vi "Draw Circle.vi"() -> ()   [LabVIEW 2016]
uses:
  Classes/Controller/Motion/A3200 Folder/A3200.lvclass
panel:
  in  "XY End":dbl[](array[numeric])=[410.0, 810.0] format="%#_13g"
  in  "Speed 2":dbl=20.0 format="%#_13g"
  in  "radius":dbl=20.0 format="%#_13g"
  in  "Direction":u16(ring)=1 items=["Clockwise", "Counter-clockwise"]
  in  "XY Center":dbl[](array[numeric])=[10.0, 0.0]
  in  "XY End 2":dbl[](array[numeric])=[400.0, 800.0]
  in  "Speed 3":dbl=20.0
  in  "Direction 2":u16(ring)=1 items=["Clockwise", "Counter-clockwise"]
  in  "Draw circle method":string(combo)="Circular"
  in  "XY":dbl[](array[numeric])=[400.0, 800.0]
  in  "Speed":dbl=40.0
  # "Circular Radius"
  # "* Draw pattern with circle radius specified, then the path would be constructed with the initial position and the end position. \n* You use this function if you don't want to calculate the circle center, you just want to draw an arc\n* You cannot draw over half circle with this function\n\n1. An arc with radius 20\n    a. radius: (20, 0)\n    b. XY End: (410, 810)"
  # "Circular"
  # "* Draw pattern with circle center specified, then the circle would be constructed with the initial position and the center position. \n* Circle Center is relative position to the initial position\n* End point could be on any position on the circle\n\n1. Full Circle with center at (410, 800)\n    a. XY Center: (10, 0)\n    b. XY End: (400, 800)\n2. Half Circle with center at (400, 810)\n    a. XY Center: (0, 10) \n    b. XY End: (400, 820)"
  # "1. This example shows how to draw a circle/arc on the XY plane  \n2. There are two methods \"Circular\" & \"Circular Radius\n3. \"Circular\" method is more commonly used \n4. Both two functions need to move gantry head to initial point of your circle/arc first"
  # "Move To Initial"
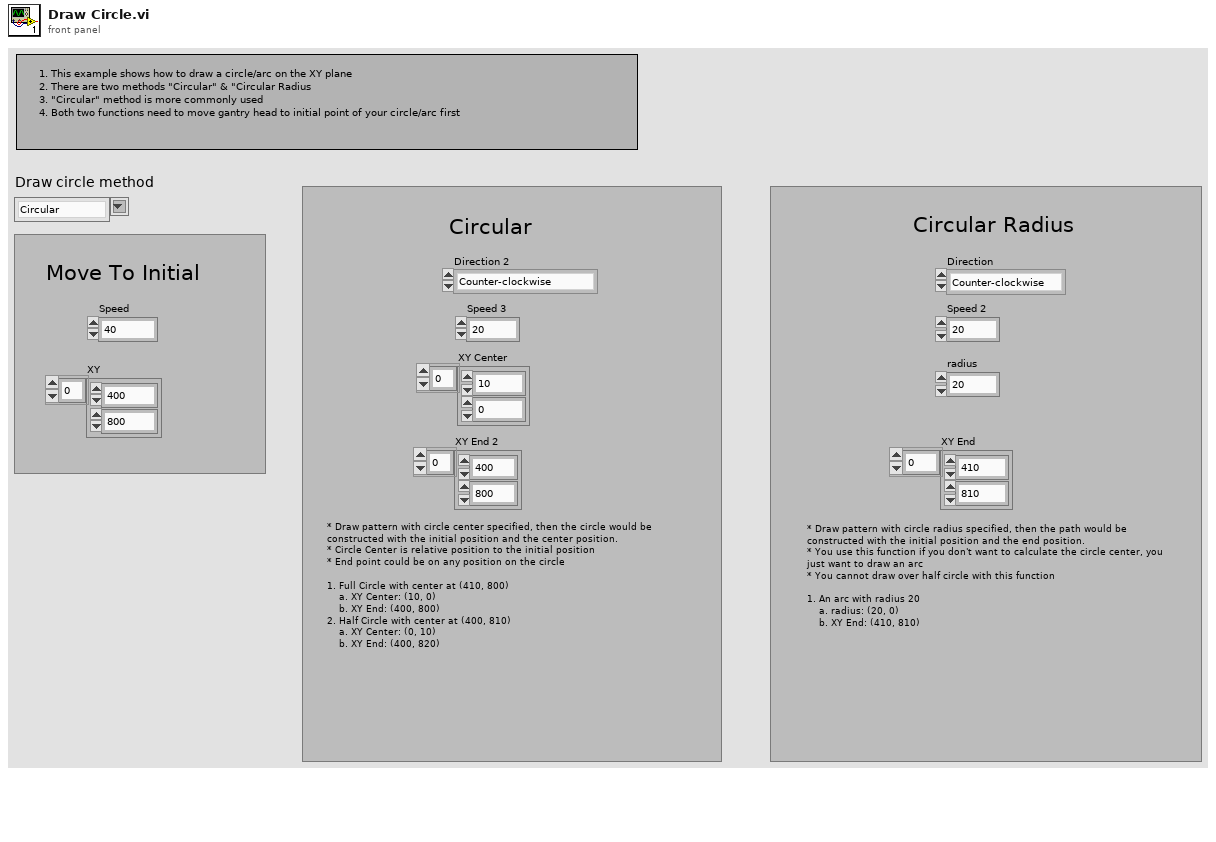
[diagram p1: front panel]
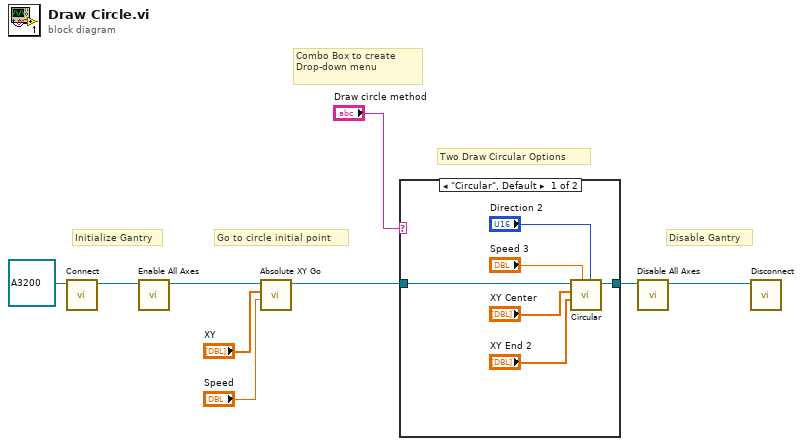
[diagram p0: block diagram]
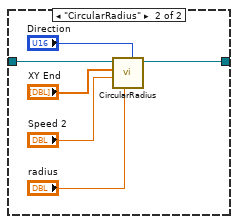
[diagram p2: hidden frame]
diagram:
  # "Disable Gantry"
  # "Go to circle initial point"
  # "Initialize Gantry"
  # "Combo Box to create Drop-down menu"
  # "Two Draw Circular Options"
  n1 = call-dynamic "Connect.vi"("Gantry in"=refnum<class "A3200.lvclass"> refnum ("A3200.lvclass")) -> ("Gantry out"=w9:refnum<class "A3200.lvclass">)  [unwired: 9 in, 1 out]
  n2 = call-dynamic "Enable All Axes.vi"("A3200 in"=w9) -> ("A3200 out"=w7:refnum<class "A3200.lvclass">)  [unwired: 9 in, 1 out]
  n3 = call-dynamic "Absolute XY Go.vi"("Speed"="Speed", "XY"="XY", "Gantry in"=w7) -> ("Gantry out"=w3:refnum<class "A3200.lvclass">)  [unwired: 7 in, 1 out]
  n4 = case shown="\"Circular\", Default" "Draw circle method" {
    tunnel: w3 -> [w15 w21]
    tunnel: [w14 w20] -> w2
    frame "Circular", Default {
      n5 = call-dynamic "Circular.vi"("Direction"="Direction 2", "Speed"="Speed 3", "XY End"="XY End 2", "XY Center"="XY Center", "Gantry in"=w15) -> ("Gantry out"=w14:refnum<class "A3200.lvclass">)  [unwired: 5 in, 1 out]
    }
    frame "CircularRadius" {
      n6 = call-dynamic "CircularRadius.vi"("Direction"="Direction", "radius"="radius", "Speed"="Speed 2", "XY End"="XY End", "A3200 in"=w21) -> ("A3200 out"=w20:refnum<class "A3200.lvclass">)  [unwired: 5 in, 1 out]
    }
  }
  n7 = call-dynamic "Disable All Axes.vi"("Gantry in"=w2) -> ("Gantry out"=w4:refnum<class "A3200.lvclass">)  [unwired: 9 in, 1 out]
  n8 = call-dynamic "Disconnect.vi"("Gantry in"=w4) -> ()  [unwired: 9 in, 1 out]
